vi "CameraInit.vi"(8 "Last Attempt":bool, 11 "IO Cluster In":T1={"Error"={"status"=FALSE, "code"=0, "source"=""}, "Encoder Calibration Values"=[22, 216], "Update Calibration"=FALSE, "JPEG Resolutions"=3, "Raw Resolutions"=1, "Image Mode"=enum."RAW Gray Scale", "FPGA Ref"=refnum} {"JPEG Resolutions" items=["160x128"=3, "320x240"=5, "640x480"=7]; "Raw Resolutions" items=["80x60"=1, "160x120"=3, "128x128"=9, "128x96"=11]}) -> (0 "Exit":bool, 1 "Sync Complete":bool, 3 "IO Cluster Out":T1={"Error"={"status"=FALSE, "code"=0, "source"=""}, "Encoder Calibration Values"=[22, 216], "Update Calibration"=FALSE, "JPEG Resolutions"=3, "Raw Resolutions"=1, "Image Mode"=enum."RAW Gray Scale", "FPGA Ref"=refnum} {"JPEG Resolutions" items=["160x128"=3, "320x240"=5, "640x480"=7]; "Raw Resolutions" items=["80x60"=1, "160x120"=3, "128x128"=9, "128x96"=11]}, 4 "Camera Configured":bool)   [LabVIEW 2019]
uses:
  QNET MS IO Cluster.ctl
  <vilib>/Utility/error.llb/Error Cluster From Error Code.vi
  <vilib>/rvi/errors/niLvFpgaAdjustHostInterfaceError.vi
  <vilib>/rvi/interface/nirviReadWriteControl/nirviReadWriteControl.xnode
  <vilib>/ErrorRing/Error Ring.xnode
  NiFpgaLv.dll
  <vilib>/rvi/interface/Simulation/niFpgaSimulationCallBeginRW.vi
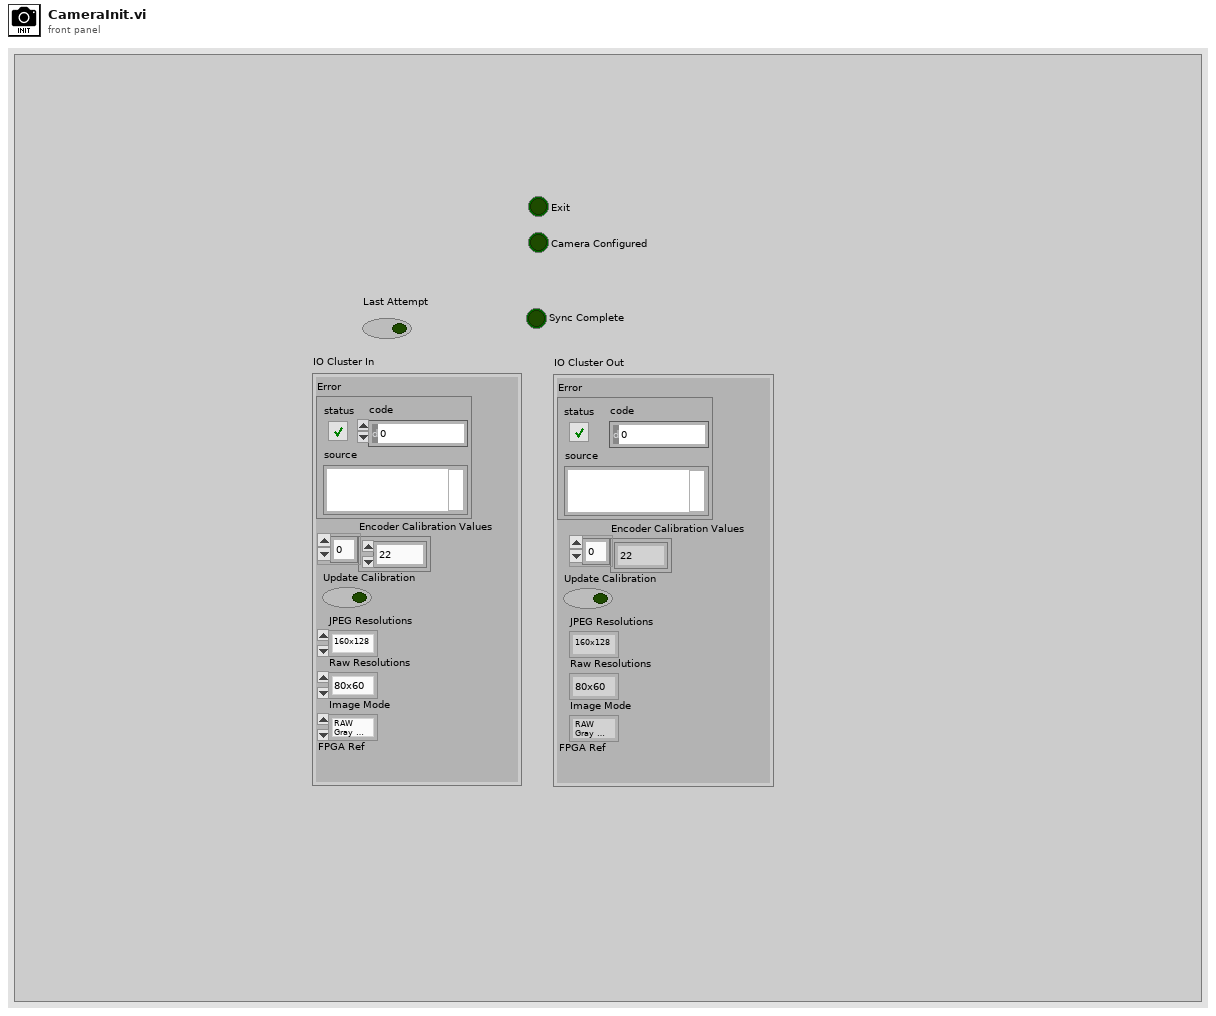
[diagram p1: front panel]
types:
  T1 = typedef "QNET MS IO Cluster.ctl" = cluster{"Error":errorcluster, "Encoder Calibration Values":i32[], "Update Calibration":bool, "JPEG Resolutions":u16, "Raw Resolutions":u16, "Image Mode":enum16{"RAW RGB", "RAW Gray Scale", "JPEG"}, "FPGA Ref":refnum<k20>}
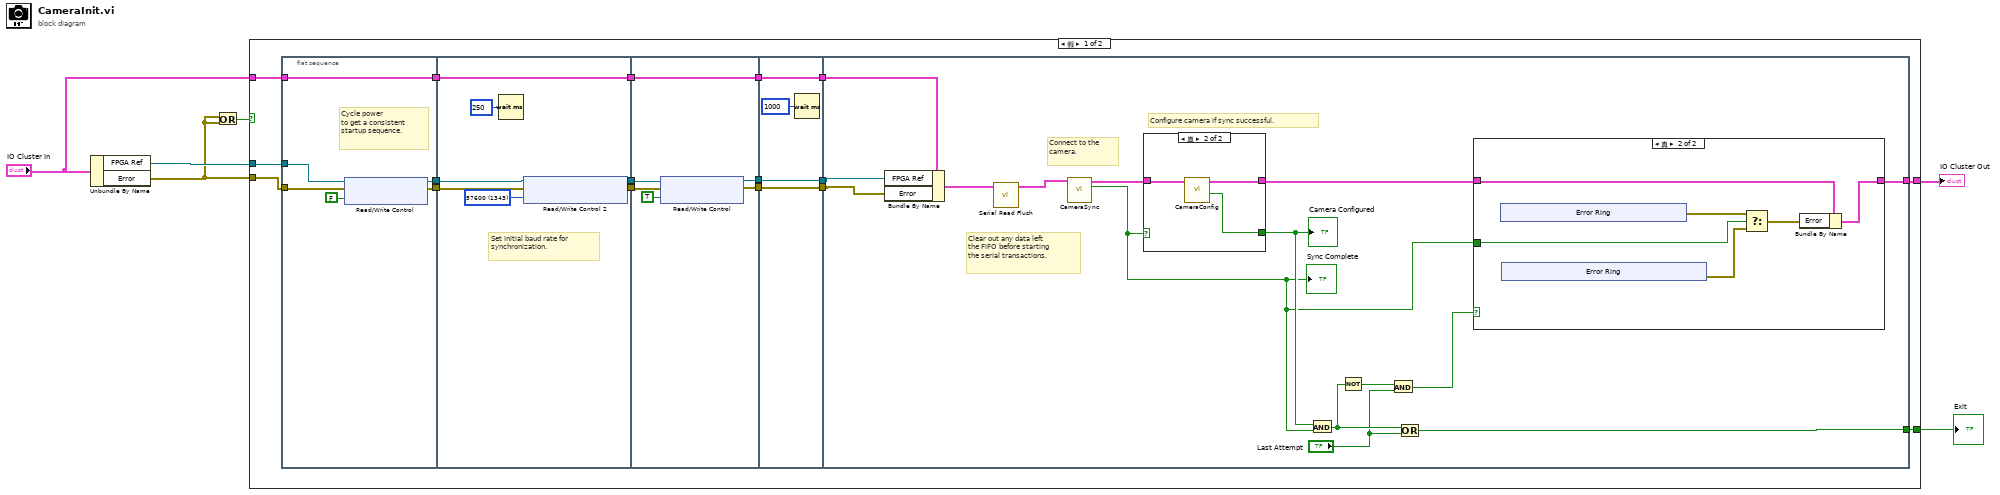
[diagram p0: block diagram]
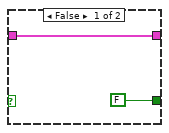
[diagram p3: hidden frame]
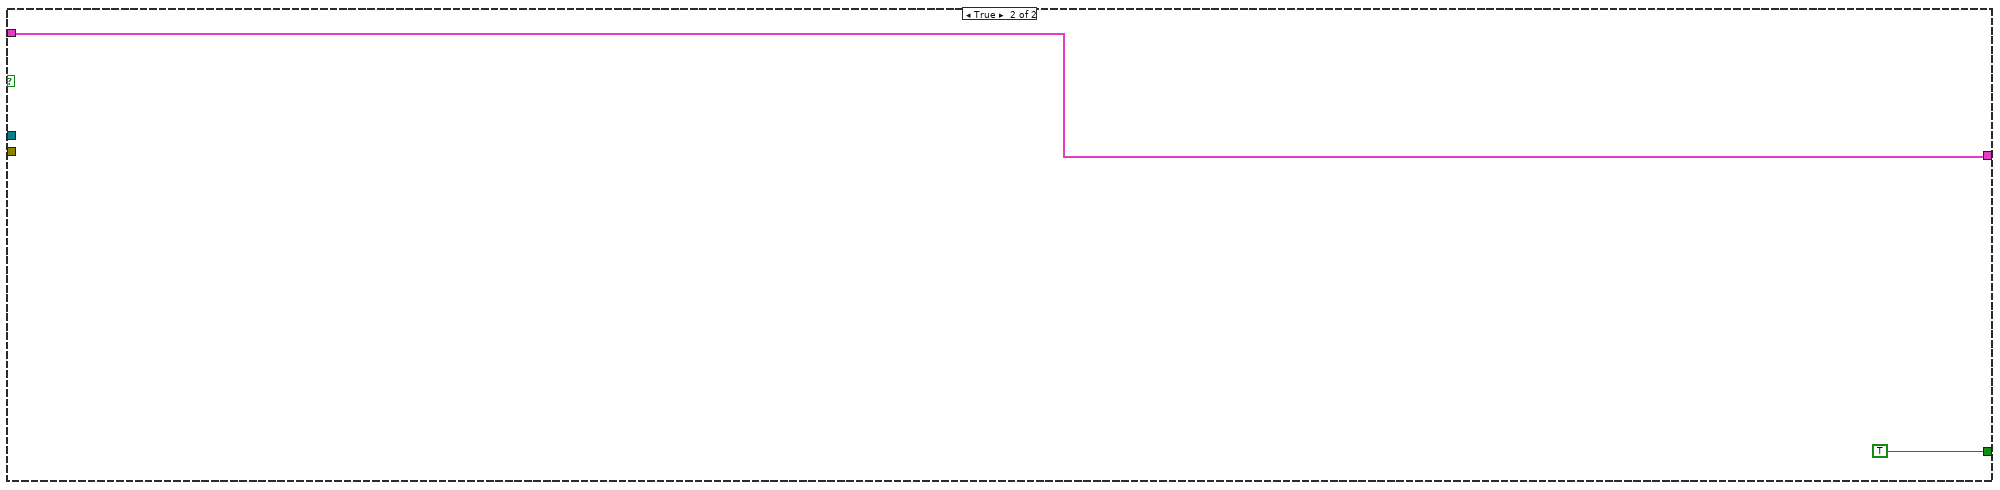
[diagram p4: hidden frame]
diagram:
  n1 = Unbundle By Name("IO Cluster In") -> ("FPGA Ref"=w6:refnum<k20>, "Error"=w4:errorcluster)
  n2 = Or(x=w4, y=w4) -> (x .or. y?=w5:bool)
  n3 = case shown="假" w5 {
    tunnel: w6 -> [w16 _]
    tunnel: w4 -> [w15 _]
    tunnel: [w14 w85] -> w2
    tunnel: "IO Cluster In" -> [w8 w85]
    tunnel: [w13 TRUE] -> w3
    frame False {
      n4 = flat-sequence {
        tunnel: w15 -> [w28]
        tunnel: w16 -> [w27]
        tunnel: [w26] -> w23
        tunnel: [w25] -> w22
        tunnel: [w24] -> w9
        tunnel: w8 -> [w24]
        tunnel: w23 -> [w31]
        tunnel: w22 -> [w30]
        tunnel: [w32] -> w21
        tunnel: [w35] -> w10
        tunnel: w9 -> [w35]
        tunnel: [w33] -> w7
        tunnel: w21 -> [w40]
        tunnel: [w39] -> w20
        tunnel: [w38] -> w19
        tunnel: [w37] -> w11
        tunnel: w10 -> [w37]
        tunnel: w7 -> [w41]
        tunnel: w20 -> [w45]
        tunnel: w19 -> [w44]
        tunnel: [w45] -> w18
        tunnel: [w44] -> w17
        tunnel: [w43] -> w12
        tunnel: w11 -> [w43]
        tunnel: w18 -> [w48]
        tunnel: w17 -> [w47]
        tunnel: [w53] -> w14
        tunnel: [w57] -> w13
        tunnel: w12 -> [w50]
        frame #0 {
          # "Cycle power\nto get a consistent\nstartup sequence."
          n5 = xnode "Read/Write Control"("FPGA VI引用输入"=w27, "错误输入"=w28, "Camera Power"=FALSE) -> ("FPGA VI引用输出"=w25:refnum<k20>, "错误输出"=w26:errorcluster)
        }
        frame #1 {
          w34 = u16 1343 items=["9600"=8063, "19200"=4031, "38400"=2015, "57600"=1343, "115200"=671, "153600"=503, "230400"=335, "460800"=167, "921600"=83, "1228800"=62, "1843200"=41, "3686400"=20] ("Baud Rate")
          # "Set initial baud rate for\nsynchronization."
          n6 = Wait (ms)(milliseconds to wait=u32 250) -> ()  [unwired: 1 out]
          n7 = xnode ("Read/Write Control 2")("FPGA VI引用输入"=w30, "错误输入"=w31, "UART Clock Divisor"=w34) -> ("FPGA VI引用输出"=w33:refnum<k20>, "错误输出"=w32:errorcluster)
        }
        frame #2 {
          n8 = xnode "Read/Write Control"("FPGA VI引用输入"=w41, "错误输入"=w40, "Camera Power"=TRUE) -> ("FPGA VI引用输出"=w39:refnum<k20>, "错误输出"=w38:errorcluster)
        }
        frame #3 {
          n9 = Wait (ms)(milliseconds to wait=u32 1000) -> ()  [unwired: 1 out]
        }
        frame #4 {
          # "Configure camera if sync successful."
          # "Connect to the\ncamera."
          # "Clear out any data left\nthe FIFO before starting\nthe serial transactions."
          n10 = Bundle By Name(cluster=w50, "FPGA Ref"=w48, "Error"=w47) -> (w60:T1)
          n11 = call "Serial Read Flush.vi"("IO Cluster In"=w60) -> ("IO Cluster Out"=w59:T1)  [unwired: 10 in]
          n12 = call "CameraSync.vi"("IO Cluster In"=w59) -> ("Sync Complete"=w51:bool, "IO Cluster Out"=w61:T1)  [unwired: 8 in, 1 out]
          "Sync Complete" <- w51
          n13 = case shown="真" w51 {
            tunnel: [w80 w83] -> w54
            tunnel: w61 -> [w80 w82]
            tunnel: [FALSE ("Configuration Complete") w81] -> w58
            frame False {
            }
            frame True {
              n14 = call "CameraConfig.vi"("IO Cluster In"=w82) -> ("Configuration Complete"=w81:bool, "IO Cluster Out"=w83:T1)  [unwired: 8 in, 1 out]
            }
          }
          "Camera Configured" <- w58
          n15 = And(x=w58, y=w51) -> (x .and. y?=w56:bool)
          n16 = Not(x=w56) -> (.not. x?=w55:bool)
          n17 = And(x=w55, y="Last Attempt") -> (x .and. y?=w52:bool)
          n18 = Or(x=w56, y="Last Attempt") -> (x .or. y?=w57:bool)
          n19 = case shown="真" w52 {
            tunnel: w54 -> [w62 w68]
            tunnel: [w62 w67] -> w53
            tunnel: w51 -> [_ w66]
            frame False {
            }
            frame True {
              n20 = xnode "Error Ring"() -> ("错误输出"=w64:errorcluster)
              n21 = xnode "Error Ring"() -> ("错误输出"=w63:errorcluster)
              n22 = Select(t=w64, s=w66, f=w63) -> (s? t:f=w65:errorcluster)
              n23 = Bundle By Name(cluster=w68, "Error"=w65) -> (w67:T1)
            }
          }
        }
      }
    }
    frame True {
    }
  }
  "Exit" <- w3
  "IO Cluster Out" <- w2
